vi "Photobleach Custom.vi"(8 "error in (no error)":errorcluster, 10 "Length (mm)":dbl, 11 "Stage Controller in":refnum<class "Stage Controller.lvclass">) -> (0 "error out":errorcluster, 3 "Stage Controller out":refnum<class "Stage Controller.lvclass">)   [LabVIEW 2018, in "Stage Controller.lvlib" / "Stage Controller.lvclass"]
uses:
  Stage Controller.lvclass
  Stage Controller.lvclass/Stage Controller.ctl
  Ti2/ti2lv/ti2lv.lvlib
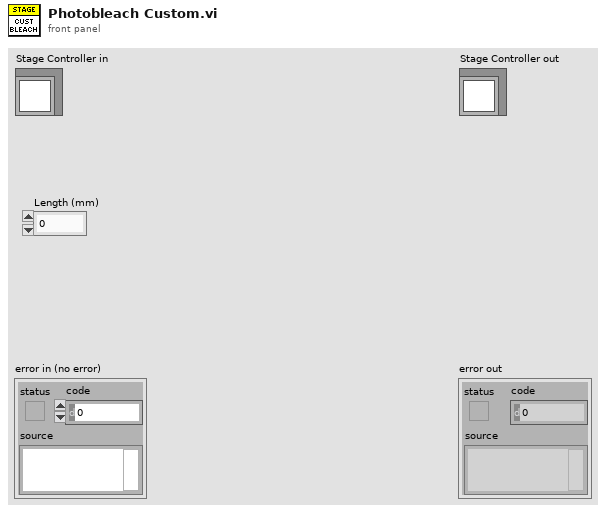
[diagram p1: front panel]
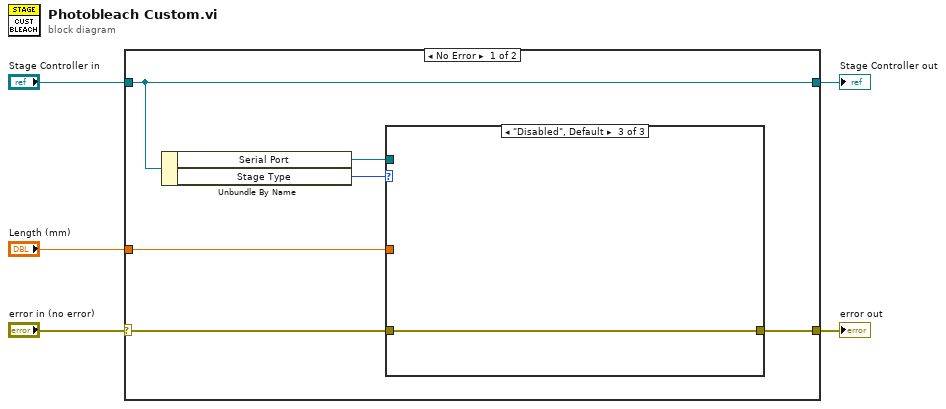
[diagram p0: block diagram]
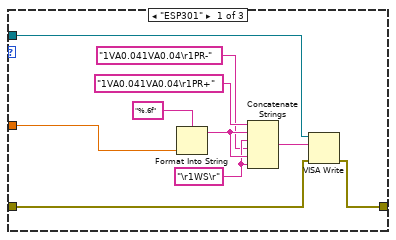
[diagram p2: hidden frame]
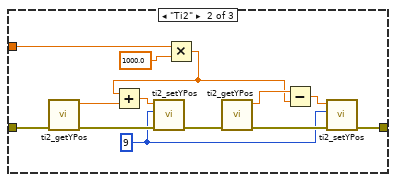
[diagram p3: hidden frame]
diagram:
  n1 = case shown="No Error" "error in (no error)" {
    selector: "error in (no error)" -> [w9 w37]
    tunnel: [w8 w37] -> w4
    tunnel: [w11 w36] -> w2
    tunnel: "Stage Controller in" -> [w11 w36]
    tunnel: "Length (mm)" -> [w10 _]
    frame No Error {
      n2 = Unbundle By Name(w11) -> ("Serial Port"=w7:refnum<visa-resource-name>, "Stage Type"=w6:enum16{"Disabled", "ESP301", "Ti2"})
      n3 = case shown="\"Disabled\", Default" w6 {
        tunnel: w10 -> [w12 w25 _]
        tunnel: w9 -> [w14 w24 w35]
        tunnel: [w15 w23 w35] -> w8
        tunnel: w7 -> [w13 _ _]
        frame "ESP301" {
          w17 = "\r1WS\r" ("write buffer")
          n4 = Format Into String(format string="%.6f", w12) -> (resulting string=w21:string)  [unwired: 2 in, 1 out]
          n5 = Concatenate Strings("1VA0.041VA0.04\r1PR+" ("write buffer"), w21, w17, "1VA0.041VA0.04\r1PR-" ("write buffer"), w21, w17) -> (w20:string)
          n6 = VISA Write(VISA resource name=w13, write buffer=w20, error in (no error)=w14) -> (error out=w15:errorcluster)  [unwired: 2 out]
        }
        frame "Ti2" {
          w22 = 9 ("speed")
          n7 = call "ti2_getYPos.vi"("error in (no error)"=w24) -> ("error out"=w34:errorcluster, "y Position (um)"=w32:dbl)  [unwired: 9 in]
          n8 = Multiply(x=w25, y=1000.0) -> (x*y=w26:dbl)
          n9 = Add(x=w26, y=w32) -> (x+y=w33:dbl)
          n10 = call "ti2_setYPos.vi"("error in (no error)"=w34, "speed"=w22, "y Position (um)"=w33) -> ("error out"=w29:errorcluster)  [unwired: 8 in]
          n11 = call "ti2_getYPos.vi"("error in (no error)"=w29) -> ("error out"=w30:errorcluster, "y Position (um)"=w27:dbl)  [unwired: 9 in]
          n12 = Subtract(x=w27, y=w26) -> (x-y=w28:dbl)
          n13 = call "ti2_setYPos.vi"("error in (no error)"=w30, "speed"=w22, "y Position (um)"=w28) -> ("error out"=w23:errorcluster)  [unwired: 8 in]
        }
        frame "Disabled", Default {
        }
      }
    }
    frame Error {
    }
  }
  "error out" <- w4
  "Stage Controller out" <- w2
